vi "checkStiffnessOutOfRange.vi"(8 "error in (no error)":errorcluster, 11 "Model in":refnum<class "Model.lvclass">) -> (0 "error out":errorcluster, 2 "stiffnessOutOfRangeIsTrue":bool, 3 "Model out":refnum<class "Model.lvclass">)   [LabVIEW 2013, in "Model.lvclass"]
uses:
  Model.lvclass
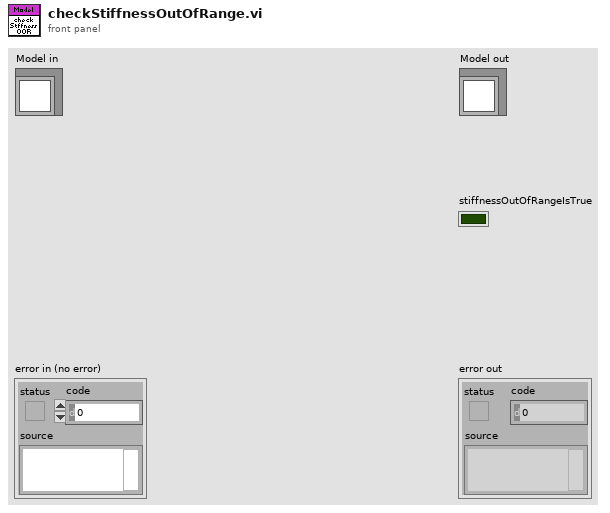
[diagram p1: front panel]
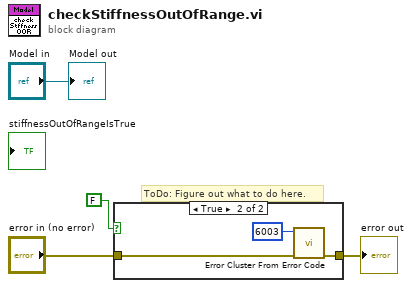
[diagram p0: block diagram]
diagram:
  # "ToDo: Figure out what to do here."
  n1 = case shown="True" FALSE {
    tunnel: "error in (no error)" -> [w5 w8]
    tunnel: [w5 w7] -> w2
    frame False {
    }
    frame True {
      n2 = call <vilib>:"Error Cluster From Error Code.vi"("error in (no error)"=w8, "error code (0)"=6003) -> ("error out"=w7:errorcluster)  [unwired: 7 in]
    }
  }
  "error out" <- w2
  "Model out" <- "Model in"
